vi "BLED1112_app-discovery scan(170203).vi"(0 "COM in":refnum<visa-resource-name>="COM8", 9 "Device List":refnum<vi>, 11 "LED ref":refnum<vi>, 12 "Stop triger ref 1":refnum<vi>, 13 "Stop triger ref 2":refnum<vi>) -> (4 "COM out":refnum<visa-resource-name>, 6 "BLED112 Dongle Info":string="Major: 1, Minor: 3, Patch: 2, Build: 122, LL ver: 3, Protocol ver: 1 and HW ver: 3  ", 10 "Scan success?":bool, 14 "Stop triger ref 1 out":bool, 15 "error out":errorcluster caption="에러 출력")   [LabVIEW 2015]
panel:
  # "BLE Discovery"
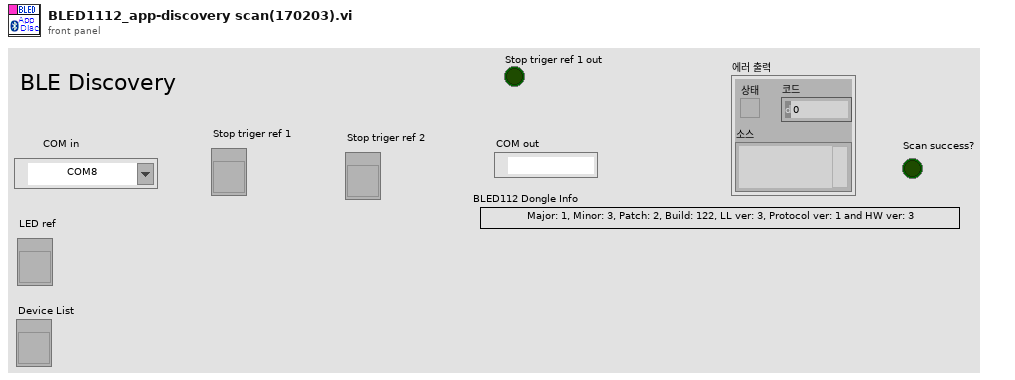
[diagram p1: front panel]
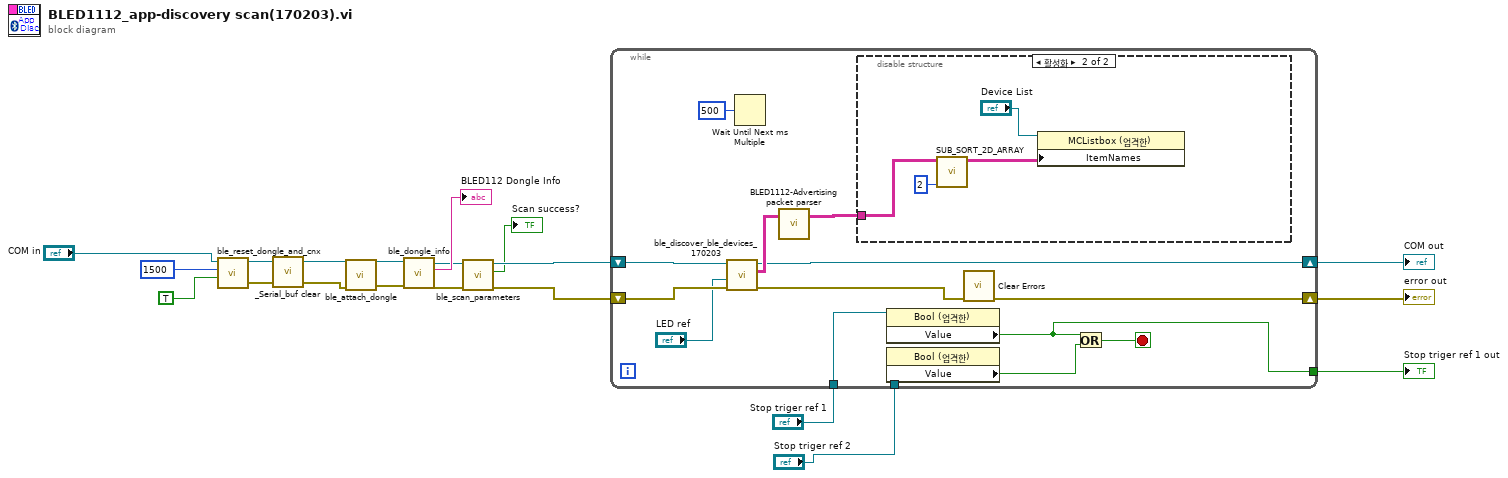
[diagram p0: block diagram]
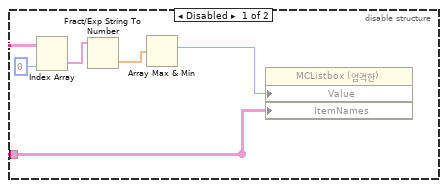
[diagram p2: hidden frame]
diagram:
  n1 = call "ble_reset_dongle_and_cnx.vi"("Reset?"=TRUE, "wait time (100)"=u32 1500, "COM Bluegiga in"="COM in") -> ("error out"=w10:errorcluster, "COM Bluegiga out"=w11:refnum<visa-resource-name>)  [unwired: 7 in]
  n2 = call "_Serial_buf clear.vi"("에러 출력 2"=w10, "Serial Port"=w11) -> ("에러 출력"=w8:errorcluster, "Serial Port 2"=w9:refnum<visa-resource-name>)  [unwired: 2 in]
  n3 = call "ble_attach_dongle.vi"("error in (no error)"=w8, "COM Bluegiga in"=w9) -> ("error out"=w13:errorcluster, "COM Bluegiga out"=w14:refnum<visa-resource-name>)  [unwired: 8 in]
  n4 = call "ble_dongle_info.vi"("error in (no error)"=w13, "COM Bluegiga in"=w14) -> ("error out"=w18:errorcluster, "info"=→"BLED112 Dongle Info":string, "COM Bluegiga out"=w19:refnum<visa-resource-name>)  [unwired: 7 in]
  n5 = call "ble_scan_parameters.vi"("error in (no error)"=w18, "COM Bluegiga in"=w19) -> ("error out"=w16:errorcluster, "success?"=→"Scan success?":bool, "COM Bluegiga out"=w17:refnum<visa-resource-name>)  [unwired: 7 in]
  n6 = while {
    shift-right: [w29] -> w4
    shift-left: w17 -> [w34]
    shift-right: [w31] -> w7
    shift-left: w16 -> [w33]
    tunnel: [w22] -> w3
    tunnel: "Stop triger ref 1" -> [w26]
    tunnel: "Stop triger ref 2" -> [w25]
    stop <- w23 stop-if-true
    n7 = call "ble_discover_ble_devices_170203.vi"("error in (no error)"=w33, "LED ref"="LED ref", "COM Bluegiga in"=w34) -> ("error out"=w28:errorcluster, "Devices"=w32:string[][], "COM Bluegiga out"=w29:refnum<visa-resource-name>)  [unwired: 6 in]
    n8 = Wait Until Next ms Multiple(millisecond multiple=u32 500 ("ms 배수")) -> ()  [unwired: 1 out]
    n9 = call "BLED1112-Advertising  packet parser.vi"("Advertising Data (in)"=w32) -> ("Advertising Data  (out)"=w21:string[][])  [unwired: 2 in]
    n10 = disable-structure shown="활성화" {
      disable-tunnel: w21 -> [w35 w44]
      frame Disabled {
        n11 = Index Array(array=w35, index (col)=0 ("비활성화된 인덱스 (열)")) -> (element=w39:string[])  [unwired: 1 in]
        n12 = Fract/Exp String To Number(string=w39) -> (number=w38:dbl[])  [unwired: 3 in, 1 out]
        n13 = Array Max & Min(array=w38) -> (max index (indices)=w36:i32)  [unwired: 3 out]
        n14 = property class="MCListbox (엄격한)"("Value"=w36, "ItemNames"=w35) -> (reference=w37:refnum<vi>)  [unwired: 1 in, 2 out]
      }
      frame Enabled {
        n15 = call "SUB_SORT_2D_ARRAY.vi"("Index sort by"=2, "array"=w44) -> ("Sorted array"=w42:string[][])  [unwired: 9 in]
        n16 = property class="MCListbox (엄격한)"(reference="Device List", "ItemNames"=w42) -> ()  [unwired: 1 in, 2 out]
      }
    }
    n17 = property class="Bool (엄격한)"(reference=w26) -> ("Value"=w22:bool)  [unwired: 1 in, 2 out]
    n18 = property class="Bool (엄격한)"(reference=w25) -> ("Value"=w24:bool)  [unwired: 1 in, 2 out]
    n19 = call <vilib>:"Clear Errors.vi"("error in (no error)"=w28) -> ("error out"=w31:errorcluster)  [unwired: 5 in, 1 out]
    n20 = Or(x=w22, y=w24) -> (x .or. y?=w23:bool)
  }
  "COM out" <- w4
  "error out" <- w7
  "Stop triger ref 1 out" <- w3
